vi "Write Matching Devices.vi"(10 "Matching Devices":string[](array[string]), 11 "Respond with Devices for Function Msg in":refnum<class "Respond with Devices for Function Msg.lvclass">) -> (3 "Respond with Devices for Function Msg out":refnum<class "Respond with Devices for Function Msg.lvclass">)   [LabVIEW 2016, in "Controller Actor.lvlib" / "Respond with Devices for Function Msg.lvclass"]
uses:
  <userlib>/Common Components/Controller/Messages/Respond with Devices for Function Msg/Respond with Devices for Function Msg.lvclass
  <userlib>/Common Components/Controller/Messages/Respond with Devices for Function Msg/Respond with Devices for Function Msg.lvclass/Respond with Devices for Function Msg.ctl
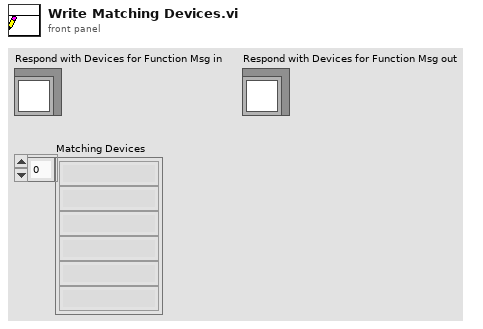
[diagram p1: front panel]
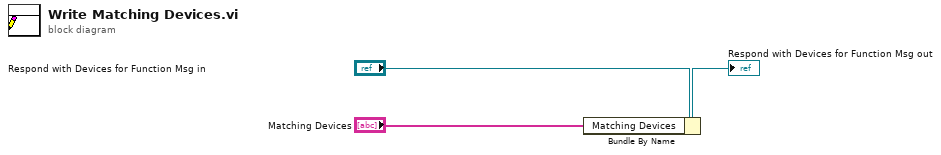
[diagram p0: block diagram]
diagram:
  n1 = Bundle By Name(cluster="Respond with Devices for Function Msg in", "Matching Devices"="Matching Devices") -> (→"Respond with Devices for Function Msg out":refnum<class "Respond with Devices for Function Msg.lvclass">)
